vi "DrawShape.vi"(8 "error in (no error)":errorcluster, 9 "Center Position in":cluster{"x":sgl, "y":sgl}, 10 "Picture in":picture, 11 "RectangleShape in":refnum<class "RectangleShape.lvclass">) -> (0 "error out":errorcluster, 2 "Picture out":picture, 3 "RectangleShape out":refnum<class "RectangleShape.lvclass">)   [LabVIEW 2022 SP3, in "RectangleShape.lvclass"]
uses:
  RectangleShape.lvclass
  RectangleShape.lvclass/RectangleShape.ctl
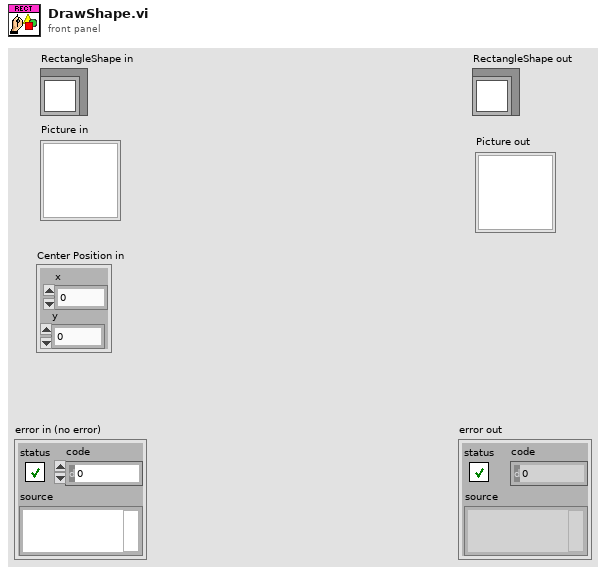
[diagram p1: front panel]
types:
  T1 = cluster{"left":i16, "top":i16, "right":i16, "bottom":i16}
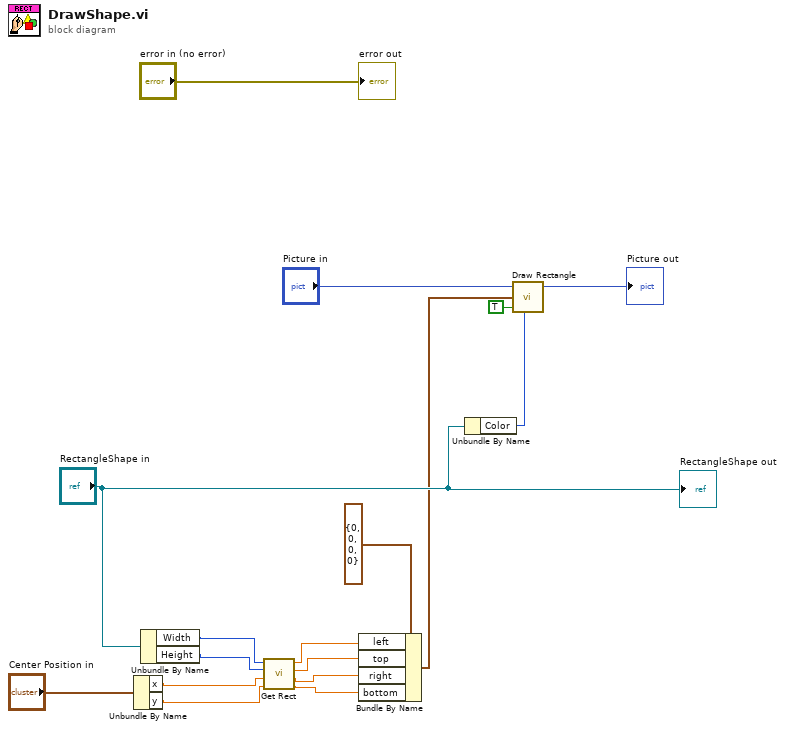
[diagram p0: block diagram]
diagram:
  n1 = Unbundle By Name("Center Position in") -> ("x"=w7:sgl, "y"=w8:sgl)
  n2 = Unbundle By Name("RectangleShape in") -> ("Width"=w5:i16, "Height"=w6:i16)
  n3 = call "Get Rect.vi"("y"=w8, "x"=w7, "Height"=w6, "Width"=w5) -> ("Bottom"=w1:sgl, "Right"=w2:sgl, "Top"=w3:sgl, "Left"=w4:sgl)
  n4 = Bundle By Name(cluster=T1 {"left"=0, "top"=0, "right"=0, "bottom"=0} ("rect"), "left"=w4, "top"=w3, "right"=w2, "bottom"=w1) -> (w10:T1)
  n5 = Unbundle By Name("RectangleShape in") -> ("Color"=w14:u32)
  n6 = call <vilib>:"Draw Rectangle.vi"("picture"="Picture in", "rect"=w10, "fill?(F)"=TRUE, "color(black)"=w14) -> ("new picture"=→"Picture out":picture)  [unwired: 5 in]
  "error out" <- "error in (no error)"
  "RectangleShape out" <- "RectangleShape in"
